vi "Get Thread.vi"(11 "Transfer Group in":refnum<class "Transfer Group.lvclass">) -> (2 "thread":i32, 3 "Transfer Group out":refnum<class "Transfer Group.lvclass">)   [LabVIEW 2021, in "DSF Core.lvlib" / "Transfer Group.lvclass"]
uses:
  Transfer Group.lvclass
  Transfer Group.lvclass/Transfer Group.ctl
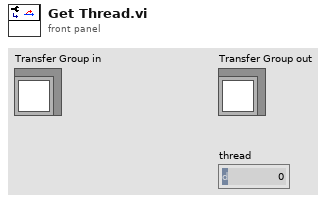
[diagram p1: front panel]
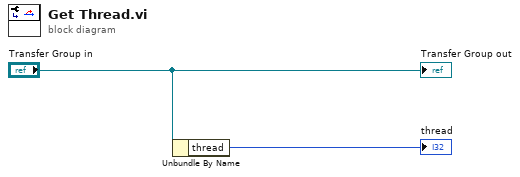
[diagram p0: block diagram]
diagram:
  n1 = Unbundle By Name("Transfer Group in") -> ("thread"=→"thread":i32)
  "Transfer Group out" <- "Transfer Group in"
